vi "Cached Name Lookup.vi"(11 "Name":string) -> (1 "Full Name":string, 2 "Success":bool, 3 "Entry ID":T1)   [LabVIEW 2017]
doc: "When it is safe to do so, this VI holds onto the latest string and ID and takes advantage of the fact that most NT access use a constant for the name. This cache avoids the name lookup."
uses:
  <vilib>/Rock Robotics/Network Tables/Field ID.ctl
  <vilib>/Rock Robotics/Network Tables/Make Table Operation.ctl
  <vilib>/Rock Robotics/Network Tables/NT Globals.vi
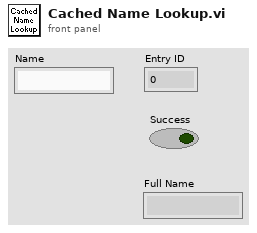
[diagram p1: front panel]
types:
  T1 = typedef "Field ID.ctl" = i32
  T2 = typedef "Make Table Operation.ctl" = enum16{"Get or Add Field", "Get Field or Add Temp", "Replace Temp ID", "Get Field ID - No Add", "Get Table Field IDs", "Get Field ID Info", "Move Field to Temp", "Validate", "Remove Field", "Remove All"}
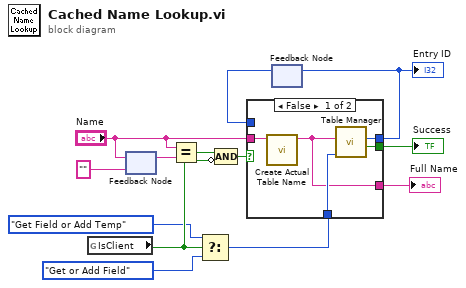
[diagram p0: block diagram]
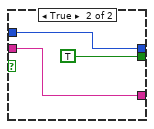
[diagram p2: hidden frame]
diagram:
  n1 = global read "NT Globals.vi" "IsClient"() -> (w13:bool)
  n2 = feedback #1("" ("Name")) -> (w6:string)
  n3 = feedback-in #1("Name") -> ()
  n4 = Equal?(x="Name", y=w6) -> (x = y?=w9:bool)
  n5 = Select(t=Make_Table_Operation."Get Field or Add Temp" ("Operation"), s=w13, f=Make_Table_Operation."Get or Add Field" ("Operation")) -> (s? t:f=w2:T2)
  n6 = Compound Arithmetic op=AND(w9, invert w13) -> (w10:bool)
  n7 = feedback #2() -> (w8:T1)  [unwired: 1 in]
  n8 = case shown="False" w10 {
    tunnel: w2 -> [w18 _]
    tunnel: [w17 TRUE ("Success")] -> w5
    tunnel: [w16 w21] -> w7
    tunnel: "Name" -> [w15 w19]
    tunnel: w8 -> [_ w21]
    tunnel: [w14 w19] -> w1
    frame False {
      n9 = call <vilib>:"Create Actual Table Name.vi"("Name or Path"=w15) -> ("Absolute Path"=w14:string)  [unwired: 10 in]
      n10 = call <vilib>:"Table Manager.vi"("Operation"=w18, "Entry Name"=w14) -> ("Success"=w17:bool, "Entry ID"=w16:T1)  [unwired: 6 in, 2 out]
    }
    frame True {
    }
  }
  "Entry ID" <- w7
  "Success" <- w5
  "Full Name" <- w1
  n11 = feedback-in #2(w7) -> ()
